vi "Create_New_Build.vi"(6 "buildSpecName":string, 7 "Programmatic? (false)":bool, 8 "error in (no error)":errorcluster, 9 "buildObject":T1, 10 "Destination Path":path, 11 "AB_Build in":refnum<class "AB_Build.lvclass">) -> (0 "error out":errorcluster, 3 "AB_Build out":refnum<class "AB_Build.lvclass">)   [LabVIEW 2020, in "AB_Build.lvclass"]
uses:
  <vilib>/AppBuilder/AB_Classes/Build/AB_Build.lvclass
  <resource>/Framework/Providers/API/ItemRef.ctl
  <vilib>/AppBuilder/AB_Classes/Source/Container/AB_Source_Container.ctl
  <vilib>/AppBuilder/AB_Exclusion_Option.ctl
  <vilib>/AppBuilder/AB_Classes/Source/AB_Source.ctl
  <vilib>/AppBuilder/AB_Source_Inclusion.ctl
  <vilib>/AppBuilder/AB_Source_Properties.ctl
  <vilib>/AppBuilder/AB_Source_Property_Type.ctl
  <vilib>/AppBuilder/AB_Classes/Source/Container/AB_Source_Container.lvclass
  e:/builds/penguin/labview/branches/2020/dev/dist/vi.lib/AppBuilder/AB_Classes/Source/AB_Source.lvclass
  <vilib>/AppBuilder/AB_Classes/Build/AB_Build.lvclass/AB_Build.ctl
  <vilib>/AppBuilder/AB_Classes/Source/AB_Source.lvclass
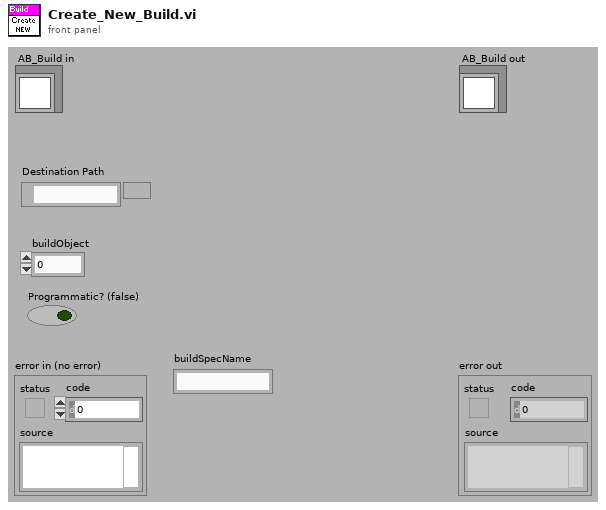
[diagram p1: front panel]
types:
  T1 = typedef "ItemRef.ctl" = u64
  T2 = typedef "AB_Source_Container.ctl" = cluster{"applyInclusion":bool, "applyDestination":bool, "applyProperties":bool, "applyPassword":bool, "applyPrefix":bool, "applySaveSetttings":bool, "dependentDestinationIndex":i32}
  T3 = cluster{"major":u16, "minor":u16, "patch":u16, "build":u16}
  T4 = typedef "AB_Exclusion_Option.ctl" = cluster{"typedefs":bool, "polymorphicVIs":bool, "unusedLibraryItems":bool, "modifyLibraryFile":bool, "edit-timeDependencies":bool, "inlineVIs":bool, "dependent PPLs":bool, "dependent DLLs":bool}
  T5 = typedef "AB_Source.ctl" = cluster{"path":path, "itemID":string, "parentIndex":i32, "sourceInclusion":T6, "destinationIndex":i32, "properties":T7[], "newName":string, "lvfile":bool, "valid":bool, "eng_inBuild":bool, "eng_isNonVILink":bool, "Amalgamation":bool, "Amalgamation Piece":bool, "eng_delimitedName":string, "preventRename":bool}
  T6 = typedef "AB_Source_Inclusion.ctl" = enum16{"IncludeIfReferenced", "Include", "Exclude", "TopLevel"}
  T7 = typedef "AB_Source_Properties.ctl" = cluster{"sourcePropertyType":T8, "value":variant}
  T8 = typedef "AB_Source_Property_Type.ctl" = enum16{"Remove block diagram", "Remove front panel", "Password", "Window has title bar", "Show menu bar", "Show vertical scroll bar", "Show horizontal scroll bar", "Show toolbar", "Show Abort button", "Show fp when called", "Window behavior", "Allow user to close window", "Window run-time position", "Run when opened", "Allow debugging", "Auto error handling", "Generate guard code", "Use stack variables", "Expression folding", "Integer only", "Inline subVI"}
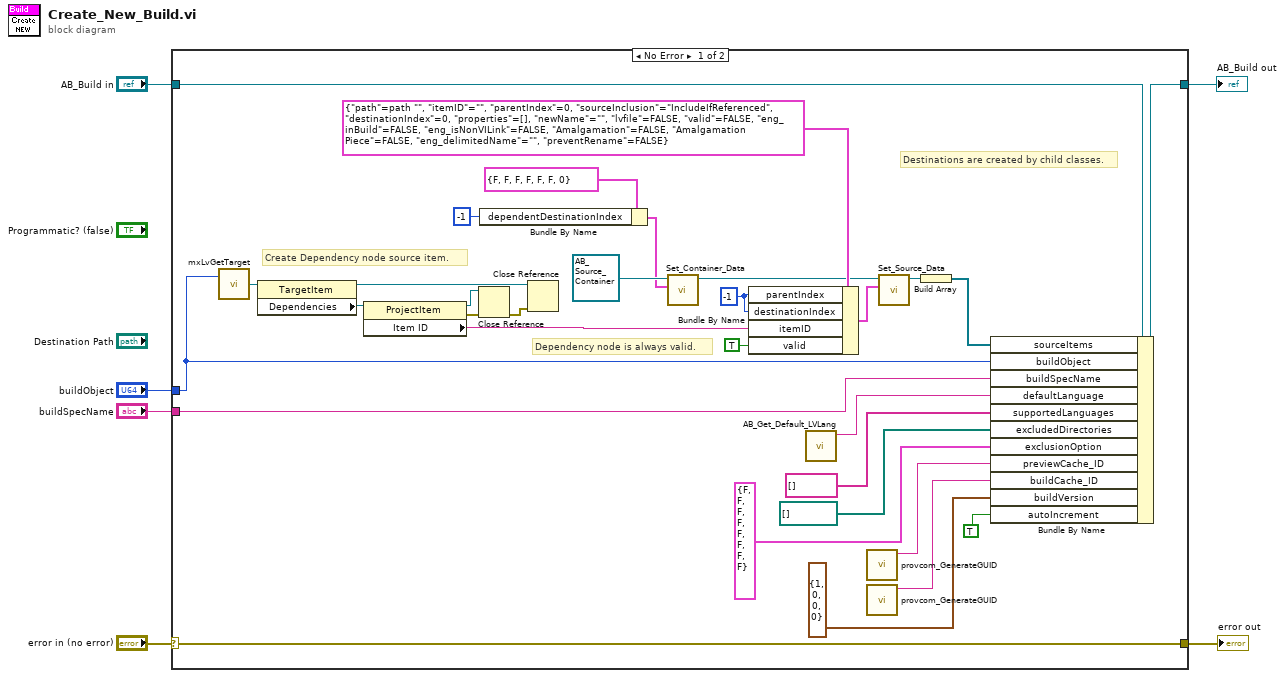
[diagram p0: block diagram]
diagram:
  n1 = case shown="No Error" "error in (no error)" {
    selector: "error in (no error)" -> [w13 w39]
    tunnel: [w13 w39] -> w5
    tunnel: [w37 w38] -> w3
    tunnel: "AB_Build in" -> [w35 w38]
    tunnel: "buildObject" -> [w14 _]
    tunnel: "buildSpecName" -> [w27 _]
    frame No Error {
      w30 = -1 ("containerIndex")
      # "Dependency node is always valid."
      # "Destinations are created by child classes."
      # "Create Dependency node source item."
      n2 = call <resource>:"mxLvGetTarget.vi"("Item"=w14) -> ("Target"=w24:refnum<vi>)  [unwired: 1 in, 2 out]
      n3 = property class="TargetItem"(reference=w24) -> (reference out=w22:refnum<vi>, "Dependencies"=w34:refnum<vi>)  [unwired: 1 in, 1 out]
      n4 = property class="ProjectItem"(reference=w34) -> (reference out=w26:refnum<vi>, error out=w25:errorcluster, "Item ID"=w31:string)  [unwired: 1 in]
      n5 = Close Reference(reference=w26, error in (no error)=w25) -> (error out=w23:errorcluster)
      n6 = Bundle By Name(cluster=T2 {"applyInclusion"=FALSE, "applyDestination"=FALSE, "applyProperties"=FALSE, "applyPassword"=FALSE, "applyPrefix"=FALSE, "applySaveSetttings"=FALSE, "dependentDestinationIndex"=0} ("data"), "dependentDestinationIndex"=-1) -> (w9:T2)
      n7 = Close Reference(reference=w22, error in (no error)=w23) -> ()  [unwired: 1 out]
      n8 = call <vilib>:"Set_Container_Data.vi"("data"=w9, "Class in"=refnum<class "AB_Source_Container.lvclass"> refnum ("AB_Container out")) -> ("Class out"=w11:refnum<class "AB_Source_Container.lvclass">)  [unwired: 8 in, 1 out]
      n9 = Bundle By Name(cluster=T5 {"path"=path "", "itemID"="", "parentIndex"=0, "sourceInclusion"=enum."IncludeIfReferenced", "destinationIndex"=0, "properties"=[], "newName"="", "lvfile"=FALSE, "valid"=FALSE, "eng_inBuild"=FALSE, "eng_isNonVILink"=FALSE, "Amalgamation"=FALSE, "Amalgamation Piece"=FALSE, "eng_delimitedName"="", "preventRename"=FALSE} ("data"), "parentIndex"=w30, "destinationIndex"=w30, "itemID"=w31, "valid"=TRUE) -> (w28:T5)
      n10 = call <vilib>:"AB_Get_Default_LVLang.vi"() -> ("env_language"=w21:string)  [unwired: 10 in, 1 out]
      n11 = call <resource>:"provcom_GenerateGUID.vi"() -> ("GUID"=w18:string)  [unwired: 10 in, 1 out]
      n12 = call <resource>:"provcom_GenerateGUID.vi"() -> ("GUID"=w17:string)  [unwired: 10 in, 1 out]
      n13 = call <vilib>:"Set_Source_Data.vi"("data"=w28, "Class in"=w11) -> ("Class out"=w29:refnum<class "AB_Source_Container.lvclass">)  [unwired: 8 in, 1 out]
      n14 = Build Array(w29) -> (w36:refnum<class "AB_Source_Container.lvclass">[])
      n15 = Bundle By Name(cluster=w35, "sourceItems"=w36, "buildObject"=w14, "buildSpecName"=w27, "defaultLanguage"=w21, "supportedLanguages"=string[] [], "excludedDirectories"=path[] [], "exclusionOption"=T4 {"typedefs"=FALSE, "polymorphicVIs"=FALSE, "unusedLibraryItems"=FALSE, "modifyLibraryFile"=FALSE, "edit-timeDependencies"=FALSE, "inlineVIs"=FALSE, "dependent PPLs"=FALSE, "dependent DLLs"=FALSE}, "previewCache_ID"=w18, "buildCache_ID"=w17, "buildVersion"=T3 {"major"=1, "minor"=0, "patch"=0, "build"=0} ("fileVersion"), "autoIncrement"=TRUE ("versionInfo.autoIncrement")) -> (w37:refnum<class "AB_Build.lvclass">)
    }
    frame Error {
    }
  }
  "error out" <- w5
  "AB_Build out" <- w3
